vi "LVFunction_Imop_Compute_PupilRegionsPositions.vi"(0 "Pupil.lvclass":refnum<class "Pupil.lvclass">, 11 "error in":errorcluster) -> (4 "Pupil.lvclass":refnum<class "Pupil.lvclass">, 6 "nb_black_regions":i32, 8 "nb_white_regions":i32, 10 "nb_regions":i32, 13 "Array 2":T1(array[cluster]), 15 "error out":errorcluster)   [LabVIEW 2020]
doc: "Compute the geometric parameters of the Legendre pupil from a cPupil input.\n\n--------------------------------------------------------------------------------\n\nPupilIn\n cPupil object.\n\nPupilOut\n cPupil object.\n\ncenter\n center coordinates.\n\nsize\n dimensions (width, height) of the square pupil detected\n\nErrorIn\n Error\nErrorOut\n Error"
uses:
  Pupil.lvclass
  LVClass_Pupil Read Pupil.vi
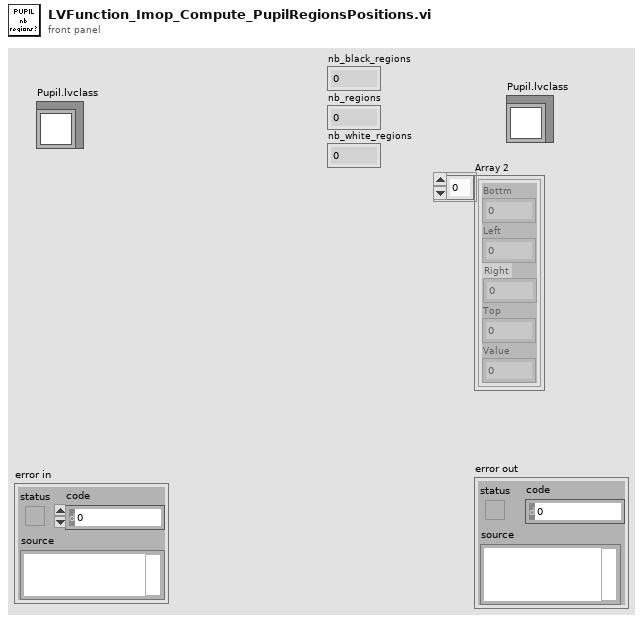
[diagram p1: front panel]
types:
  T1 = cluster{"Bottm":i32, "Left":i32, "Right":i32, "Top":i32, "Value":i32}[]
  T2 = typedef "ClassID.ctl" = i64
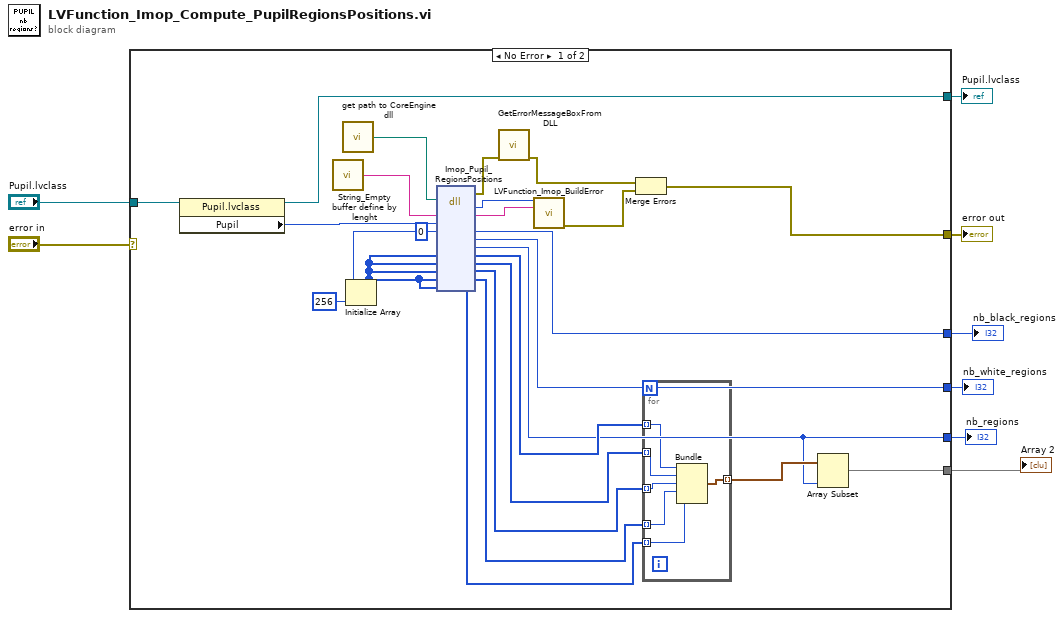
[diagram p0: block diagram]
diagram:
  n1 = case shown="No Error" "error in" {
    selector: "error in" -> [_ w40]
    tunnel: "Pupil.lvclass" -> [w23 w39]
    tunnel: [w31 w40] -> w6
    tunnel: [w22 w39] -> w5
    tunnel: [w21 _] -> w4
    tunnel: [w10 _] -> w3
    tunnel: [w20 _] -> w2
    tunnel: [w9 _] -> w1
    frame No Error {
      w18 = 0 ("nb_black_regions")
      n2 = property class="Pupil.lvclass"(reference=w23) -> (reference out=w22:refnum<class "Pupil.lvclass">, "Pupil"=w32:T2)  [unwired: 1 in, 1 out]
      n3 = call "String_Empty buffer define by lenght.vi"() -> ("Empty buffer"=w30:string)  [unwired: 1 in]
      n4 = call "get path to CoreEngine dll.vi"() -> ("path to wavekit library"=w27:path)  [unwired: 14 in, 1 out]
      n5 = Initialize Array(w18, 256 ("dimension size")) -> (w12:i32[])
      n6 = dll-call lib="D:/FLE/0.Code/CoreEngine4_Suite/LV2011_interface/DLLs/c_interface_vc100.dll" fn="Imop_Pupil_RegionsPositions"(path in=w27, "message"=w30, "Pupil"=w32, "nb_black_regions"=w18, "bottoms"=w12, "lefts"=w12, "rights"=w12, "tops"=w12, "arg10"=w12) -> (error out=w26:errorcluster, "return type"=w28:i32, "message"=w29:string, "nb_black_regions"=w21:i32, "nb_white_regions"=w20:i32, "nb_regions"=w10:i32, "bottoms"=w17:i32[], "lefts"=w16:i32[], "rights"=w15:i32[], "tops"=w14:i32[], "arg10"=w11:i32[])  [unwired: 5 in, 1 out]
      n7 = call "GetErrorMessageBoxFromDLL.vi"("error IN"=w26) -> ("error OUT"=w25:errorcluster)  [unwired: 10 in]
      n8 = call "LVFunction_Imop_BuildError.vi"("code"=w28, "String to Prepend to source (\"\")"=w29) -> ("error out"=w24:errorcluster)  [unwired: 13 in]
      n9 = Merge Errors(w25, w24) -> (w31:errorcluster)
      n10 = for {
        tunnel: w17 -> [w38] mode=indexing
        tunnel: w16 -> [w37] mode=indexing
        tunnel: w15 -> [w36] mode=indexing
        tunnel: w14 -> [w35] mode=indexing
        tunnel: [w34] -> w13 mode=indexing
        tunnel: w11 -> [w33] mode=indexing
        n11 = Bundle(w38, w37, w36, w35, w33) -> (w34:cluster{i32, i32, i32, i32, i32})  [unwired: 1 in]
      }
      n12 = Array Subset(array=w13, length=w10) -> (w9:cluster{i32, i32, i32, i32, i32}[])  [unwired: 1 in]
    }
    frame Error {
    }
  }
  "error out" <- w6
  "Pupil.lvclass" <- w5
  "nb_black_regions" <- w4
  "nb_regions" <- w3
  "nb_white_regions" <- w2
  "Array 2" <- w1
